vi "Query Questionable Data Register.vi"(8 "error in (no error)":errorcluster, 11 "VISA resource name":refnum<visa-resource-name>) -> (0 "error out":errorcluster, 2 "Questionable Data Message":string, 3 "VISA resource name out":refnum<visa-resource-name>)   [LabVIEW 2020, in "Agilent 3458.lvlib"]
doc: "Querys the data register for any alarms that may have been activated during the course of taken measurements. Specifically this VI checks to see if the HI/LOW limit register was activated by a certain measurement.\n\n<B>Note:</B> Use this VI only with other low-level VIs. The high-level VIs automatically incorporate this functionality. This VI does not check the instrument status. If you want to check the instrument status, call the Error Query VI at the conclusion of the sequence."
uses:
  Agilent 3458.lvlib
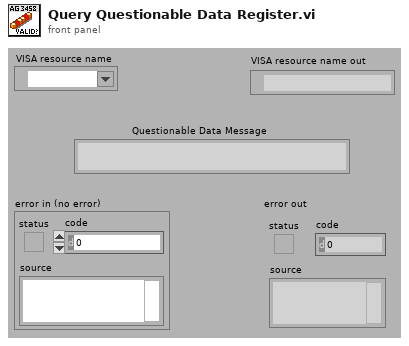
[diagram p1: front panel]
types:
  T1 = cluster{"Boolean array[0]":bool, "Boolean array[1]":bool, "Boolean array[2]":bool, "Boolean array[3]":bool, "Boolean array[4]":bool, "Boolean array[5]":bool, "Boolean array[6]":bool, "Boolean array[7]":bool, "Boolean array[8]":bool, "Boolean array[9]":bool, "Boolean array[10]":bool, "Boolean array[11]":bool, "Boolean array[12]":bool, "Boolean array[13]":bool, "Boolean array[14]":bool, "Boolean array[15]":bool}
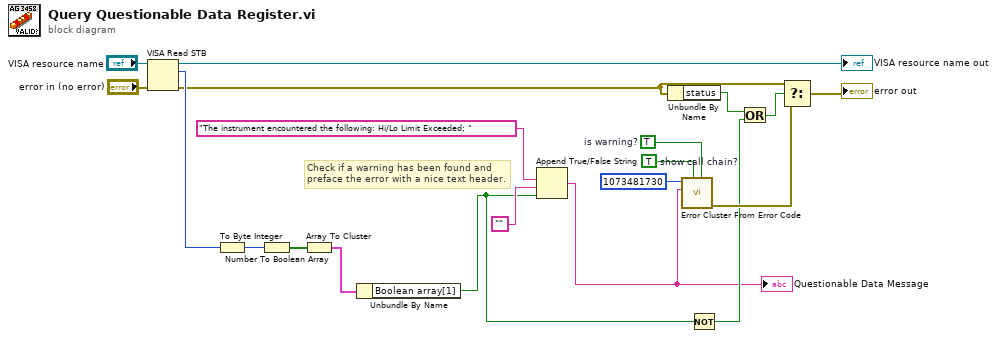
[diagram p0: block diagram]
diagram:
  w10 = TRUE  # is warning?
  w11 = TRUE  # show call chain?
  # "Check if a warning has been found and preface the error with a nice text header."
  n1 = VISA Read STB(8:"error in (no error)", 11:"VISA resource name") -> (0:w15:errorcluster, 2:w20:u16, 3:→"VISA resource name out":refnum<visa-resource-name>)
  n2 = To Byte Integer(number=w20) -> (8bit integer=w19:i8)
  n3 = Number To Boolean Array(number=w19) -> (Boolean array=w18:bool[])
  n4 = Array To Cluster(array=w18) -> (cluster=w5:T1)
  n5 = Unbundle By Name(w5) -> ("Boolean array[1]"=w4:bool)
  n6 = Append True/False String(1:w4, 2:"" ("Empty String Constant"), 3:"The instrument encountered the following: Hi/Lo Limit Exceeded; " ("true string")) -> (0:w3:string)  [unwired: 1 in]
  "Questionable Data Message" <- w3
  n7 = Unbundle By Name(w15) -> ("status"=w14:bool)
  n8 = call <vilib>:"Error Cluster From Error Code.vi"("is warning? (False)"=w10, "show call chain? (False)"=w11, "error message (\"\")"=w3, "error code (0)"=1073481730 ("t")) -> ("error out"=w9:errorcluster)  [unwired: 5 in]
  n9 = Not(x=w4) -> (.not. x?=w8:bool)
  n10 = Or(x=w14, y=w8) -> (x .or. y?=w13:bool)
  n11 = Select(t=w15, s=w13, f=w9) -> (s? t:f=→"error out":errorcluster)
